vi "[RE Python] Build Fabric of Claims.vi"(8 "Error In":errorcluster, 10 "Debugging":bool=TRUE, 11 "Split String":string[][](array[string])=[["1", "1", "3", "4", "4"], ["2", "3", "1", "4", "4"], ["3", "5", "5", "2", "2"]]) -> (0 "Error Out":errorcluster, 3 "Fabric":i32[][](array[numeric]))   [LabVIEW 2019]
doc: "After parsing Elf Claims, use each claim to update a 2D array representing the claims. Each entry in the 2D array contains an int representing the number of claims that contain it.\n\nIf Debugging is enabled and no data is passed in, then it'll use the example from the site."
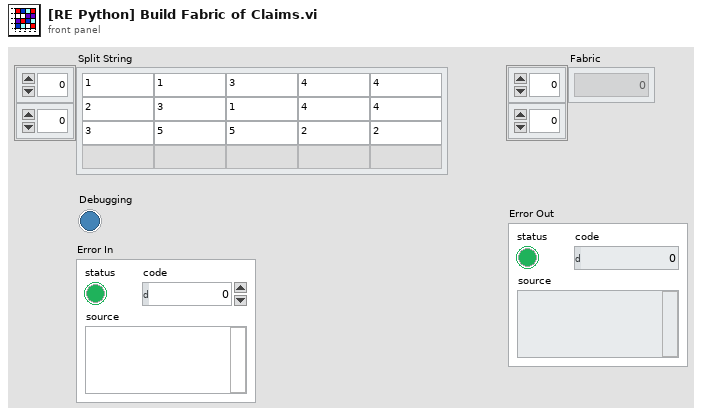
[diagram p1: front panel]
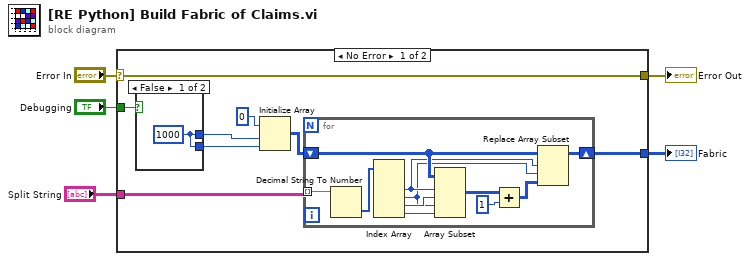
[diagram p0: block diagram]
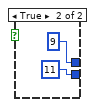
[diagram p2: hidden frame]
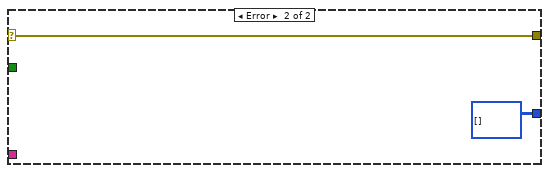
[diagram p3: hidden frame]
diagram:
  n1 = case shown="No Error" "Error In" {
    selector: "Error In" -> [w8 w29]
    tunnel: "Debugging" -> [w11 _]
    tunnel: [w8 w29] -> w3
    tunnel: [w7 i32[][] []] -> w2
    tunnel: "Split String" -> [w6 _]
    frame No Error {
      n2 = case shown="False" w11 {
        tunnel: [w14 9] -> w10
        tunnel: [w14 11] -> w9
        frame False {
          w14 = 1000
        }
        frame True {
        }
      }
      n3 = Initialize Array(0 ("element"), w10, w9) -> (w13:i32[][])
      n4 = for {
        tunnel: w6 -> [w27] mode=indexing
        shift-right: [w19] -> w7
        shift-left: w13 -> [w21]
        n5 = Decimal String To Number(string=w27) -> (number=w26:i32[])  [unwired: 2 in, 1 out]
        n6 = Index Array(array=w26) -> (element #2=w20:i32, element #3=w18:i32, element #4=w25:i32, element #5=w24:i32)  [unwired: 5 in, 1 out]
        n7 = Array Subset(array=w21, index (row)=w20, length (row)=w25, index (col)=w18, length (col)=w24) -> (w23:i32[][])
        n8 = Add(x=w23, y=1) -> (x+y=w17:i32[][])
        n9 = Replace Array Subset(array=w21, new element=w17, index (row)=w20, index (col)=w18) -> (w19:i32[][])
      }
    }
    frame Error {
    }
  }
  "Error Out" <- w3
  "Fabric" <- w2
